vi "Init.vi"(8 "error in (no error)":errorcluster caption="entrée d'erreur (pas d'erreur)", 11 "Class DIO (Default) en entrée":refnum<class "Class DIO NI.lvclass">) -> (0 "error out":errorcluster caption="sortie d'erreur", 3 "Class DIO (Default) en sortie":refnum<class "Class DIO NI.lvclass">)   [LabVIEW 2020, in "Library Instrument & Equipement.lvlib" / "Library DIO.lvlib" / "Class DIO NI.lvclass"]
uses:
  Class DIO NI.lvclass
  C:/Users/ngarcin/OneDrive - Altyor/Standard TB/Class/DIO/Class DIO (Default)/Class DIO (Default).lvclass
  <vilib>/DAQmx/create/channels.llb/DAQmx Create Channel (DO-Digital Output).vi
  <vilib>/DAQmx/create/channels.llb/DAQmx Create Channel (DI-Digital Input).vi
  Class DIO NI.lvclass/Class DIO NI.ctl
  C:/Program Files (x86)/National Instruments/LabVIEW 2020/resource/objmgr/daqmx.rc
  Commun VI/Library Commun.lvlib
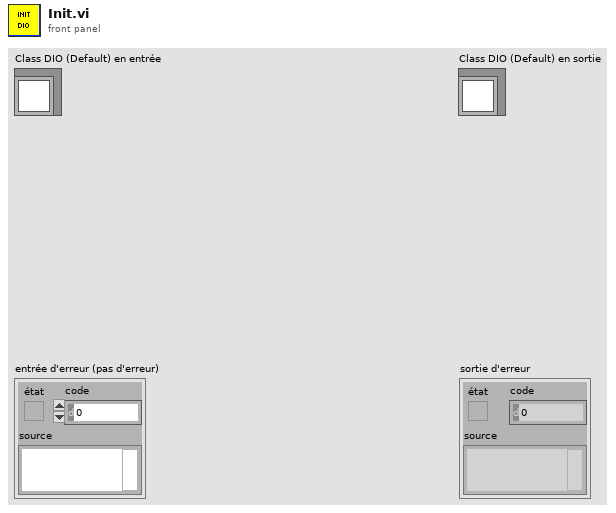
[diagram p1: front panel]
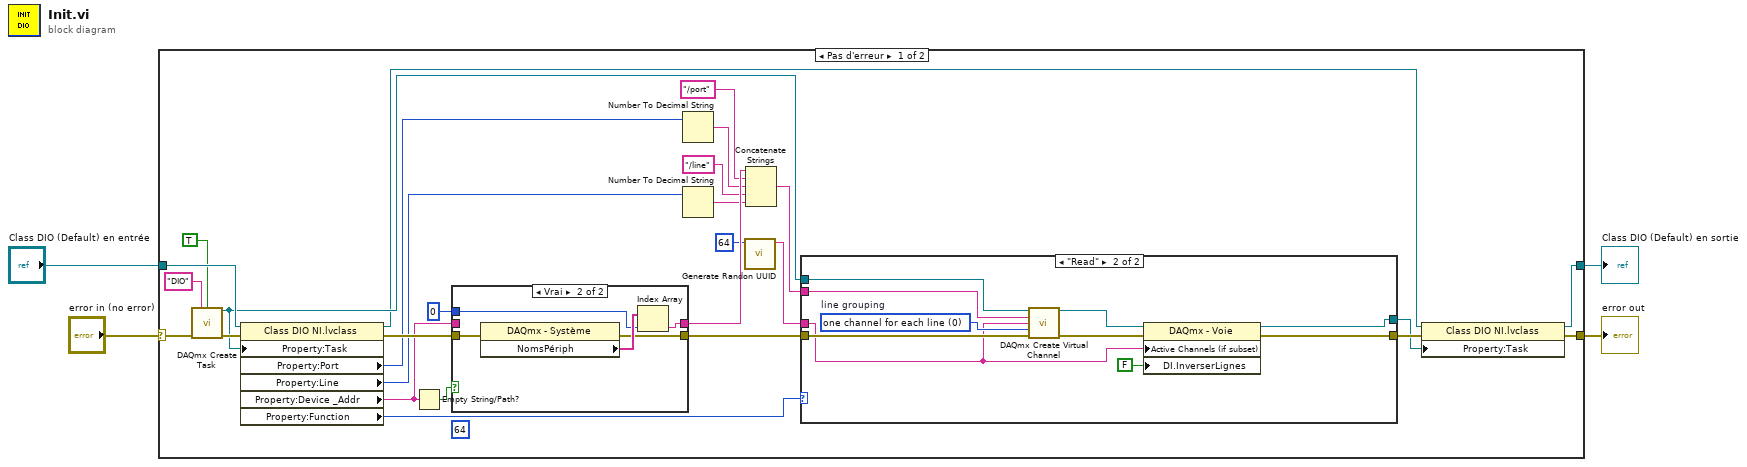
[diagram p0: block diagram]
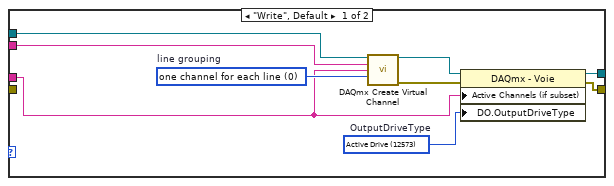
[diagram p3: hidden frame]
diagram:
  n1 = case shown="Pas d'erreur" "error in (no error)" {
    selector: "error in (no error)" -> [w30 w59]
    tunnel: [w9 w59] -> w3
    tunnel: [w8 w58] -> w1
    tunnel: "Class DIO (Default) en entrée" -> [w31 w58]
    frame No Error {
      (unwired) 64 ("Taille")
      n2 = call <vilib>:"DAQmx Create Task.vi"("new task name"="DIO", "auto cleanup"=TRUE, "error in"=w30) -> ("task out"=w28:refnum<k21>, "error out"=w29:errorcluster)  [unwired: 11 in]
      n3 = property class="Class DIO NI.lvclass"(reference=w31, error in=w29, "Property:Task"=w28) -> (reference out=w11:refnum<class "Class DIO NI.lvclass">, error out=w26:errorcluster, "Property:Port"=w23:u8, "Property:Line"=w18:u8, "Property:Device _Addr"=w13:string, "Property:Function"=w12:enum16{"Write", "Read"})
      n4 = Empty String/Path?(string/path=w13) -> (empty?=w14:bool)
      n5 = case shown="Vrai" w14 {
        tunnel: 0 ("indice") -> [_ w37]
        tunnel: w26 -> [w33 w36]
        tunnel: [w33 w35] -> w25
        tunnel: [w32 w34] -> w22
        tunnel: w13 -> [w32 _]
        frame False {
        }
        frame True {
          n6 = property class="DAQmx - Système"(error in=w36) -> (error out=w35:errorcluster, "NomsPériph"=w38:tag[])  [unwired: 1 in, 1 out]
          n7 = Index Array(array=w38, index=w37) -> (element=w34:tag)
        }
      }
      n8 = Number To Decimal String(number=w23) -> (decimal integer string=w20:string)  [unwired: 1 in]
      n9 = Number To Decimal String(number=w18) -> (decimal integer string=w17:string)  [unwired: 1 in]
      n10 = call "Generate Randon UUID.vi"("Taille"=64) -> ("chaîne"=w24:string)  [unwired: 10 in]
      n11 = Concatenate Strings(w22, "/port" ("chaîne"), w20, "/line" ("chaîne"), w17) -> (w16:string)
      n12 = case shown="\"Read\"" w12 {
        tunnel: w28 -> [w41 w56]
        tunnel: w25 -> [_ w55]
        tunnel: w24 -> [w43 w49]
        tunnel: w16 -> [w40 w54]
        tunnel: [w42 w50] -> w10
        tunnel: [w39 w48] -> w7
        frame "Write", Default {
          w45 = 12573 items=["Active Drive"=12573, "Open Collector"=12574]  # OutputDriveType
          w44 = 0 items=["one channel for each line", "one channel for all lines"]  # line grouping
          n13 = call-poly <vilib>:"DAQmx Create Virtual Channel.vi"("task in"=w41, "lines"=w40, "name to assign"=w43, "line grouping"=w44) -> ("task out"=w47:refnum<k21>, "error out"=w46:errorcluster)  [unwired: 10 in]
          n14 = property class="DAQmx - Voie"(reference=w47, error in=w46, "Active Channels (if subset)"=w43, "DO.OutputDriveType"=w45) -> (reference out=w39:refnum<k21>, error out=w42:errorcluster)
        }
        frame "Read" {
          w57 = 0 items=["one channel for each line", "one channel for all lines"]  # line grouping
          n15 = call-poly <vilib>:"DAQmx Create Virtual Channel.vi"("task in"=w56, "lines"=w54, "name to assign"=w49, "line grouping"=w57, "error in"=w55) -> ("task out"=w52:refnum<k21>, "error out"=w51:errorcluster)  [unwired: 9 in]
          n16 = property class="DAQmx - Voie"(reference=w52, error in=w51, "Active Channels (if subset)"=w49, "DI.InverserLignes"=FALSE) -> (reference out=w48:refnum<k21>, error out=w50:errorcluster)
        }
      }
      n17 = property class="Class DIO NI.lvclass"(reference=w11, error in=w10, "Property:Task"=w7) -> (reference out=w8:refnum<class "Class DIO NI.lvclass">, error out=w9:errorcluster)
    }
    frame Error {
    }
  }
  "error out" <- w3
  "Class DIO (Default) en sortie" <- w1
